vi "serialize.vi"() -> (0 "failure out":T1 {"code" format="%.0x"}, 3 "LabVIEW Text":string)   [LabVIEW 2013]
uses:
  errors/failure.ctl
  errors/severity.ctl
  <vilib>/addons/JSON API/Variant JSON/Variant to JSON.vi
  <vilib>/addons/JSON API/JSON Value/Get as JSON string (pretty).vi
  <vilib>/addons/JSON API/Get Polymorphic/JSON GetSet.lvlib
  errors/failure.lvlib
  <vilib>/addons/JSON API/Variant JSON/Variant JSON.lvlib
  <vilib>/addons/JSON API/JSON Value/JSON Value.lvclass
panel:
  in  "bool1":bool=TRUE
  in  "Time Stamp":timestamp=timestamp(3523589884.3778296 s since 1904-01-01)
  in  "num":dbl=34.0
  in  "strings":string="asdassasd"
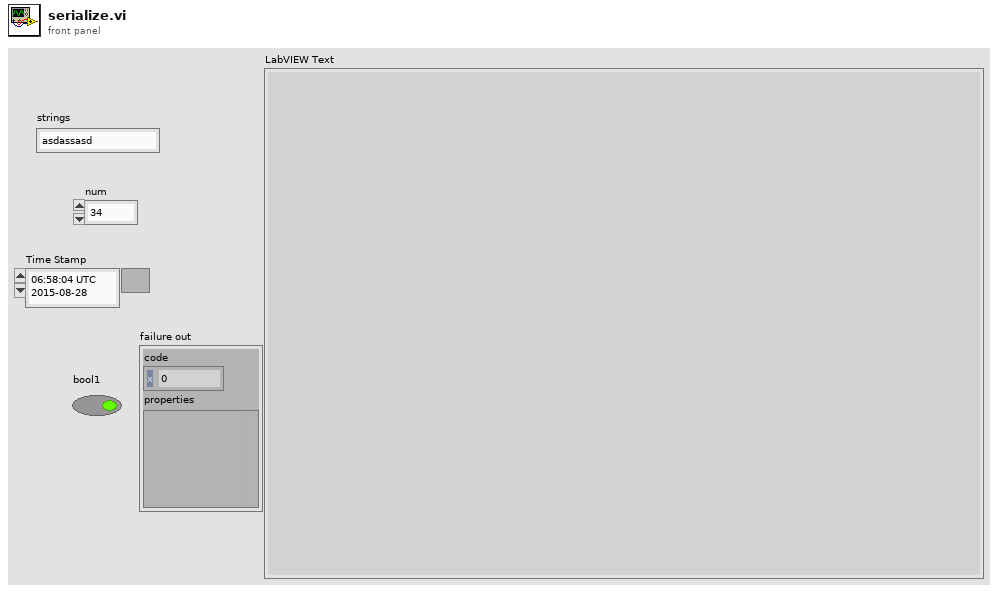
[diagram p1: front panel]
types:
  T1 = typedef "failure.lvlib/failure.ctl" = cluster{"code":i32, "properties":variant}
  T2 = typedef "failure.lvlib/severity.ctl" = enum8{"unspecified", "informational", "operation failed", "data corruption", "system corruption", "critical unknown state"}
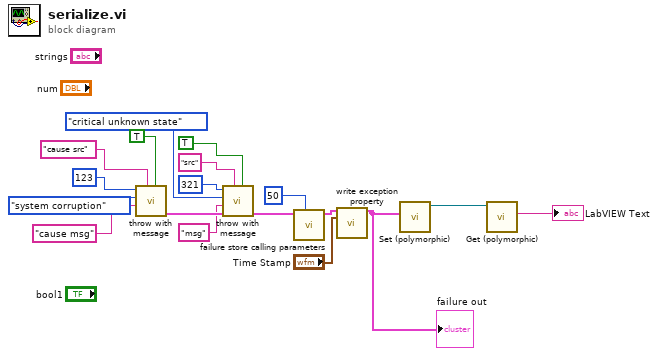
[diagram p0: block diagram]
diagram:
  n1 = call "throw with message.vi"("call chain?"=TRUE, "source"="cause src", "message"="cause msg", "severity"=severity."system corruption", "code"=123) -> ("failure out"=w10:T1)  [unwired: 6 in]
  n2 = call "throw with message.vi"("call chain?"=TRUE, "source"="src", "failure in"=w10, "message"="msg", "severity"=severity."critical unknown state", "code"=321) -> ("failure out"=w7:T1)  [unwired: 5 in]
  n3 = call "failure store calling parameters.vi"("levels"=u8 50, "failure in"=w7) -> ("failure out"=w5:T1)  [unwired: 9 in]
  n4 = call "write exception property.vi"("failure in"=w5, "Value"="Time Stamp") -> ("failure out"=w3:T1)  [unwired: 12 in, 1 out]
  "failure out" <- w3
  n5 = call-poly <vilib>:"Set (polymorphic).vi"("Variant"=w3) -> ("JSON Value out"=w9:refnum<class "JSON Value.lvclass">)  [unwired: 9 in, 1 out]
  n6 = call-poly <vilib>:"Get (polymorphic).vi"("JSON Value in"=w9) -> ("String"=→"LabVIEW Text":string)  [unwired: 9 in, 1 out]
